vi "Define.vi"(11 "Relation Definition":T1) -> (3 "Entity out":refnum<class "Entity C.lvclass">)   [LabVIEW 2022 SP3, in "Conditum.lvlib" / "Columns.lvlib" / "Entity C.lvclass"]
uses:
  Entity C.lvclass
  Entity C.lvclass/Entity C.ctl
  Relation/Relation.lvclass
  C:/dev/lv/illuminated-g/lv-conditum/Conditum/Columns/Relation/Relation.lvclass
  C:/dev/lv/illuminated-g/lv-conditum/Conditum/Columns/Type/Type.lvclass
  C:/dev/lv/illuminated-g/lv-conditum/Conditum/Columns/Entity/Entity C.lvclass
  Relation Mapping.ctl
  Conditum.lvlib
  Relation/Relation Info.ctl
  Relation/Relation Definition.ctl
  Type/Definition.ctl
  Type/Type.lvclass
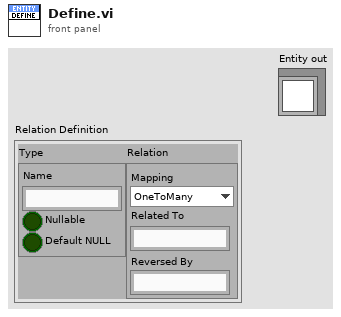
[diagram p1: front panel]
types:
  T1 = typedef "Conditum.lvlib/Columns.lvlib/Relation.lvclass/Relation Definition.ctl" = cluster{"Type":T2, "Relation":T3}
  T2 = typedef "Conditum.lvlib/Columns.lvlib/Type.lvclass/Definition.ctl" = cluster{"Name":string, "Nullable":bool, "Default NULL":bool}
  T3 = typedef "Conditum.lvlib/Relation Info.ctl" = cluster{"Mapping":T4, "Related To":string, "Reversed By":string}
  T4 = typedef "Conditum.lvlib/Relation Mapping.ctl" = enum16{"OneToMany", "ManyToOne", "ManyToMany", "OneToOne"}
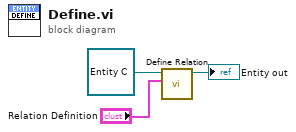
[diagram p0: block diagram]
diagram:
  n1 = call "Define Relation.vi"("Relation Definition"="Relation Definition", "Relation in"=refnum<class "Entity C.lvclass"> refnum ("Entity out")) -> ("Relation out"=→"Entity out":refnum<class "Entity C.lvclass">)  [unwired: 9 in]
